vi "Calculate Color Index Array.vi"(8 "error in (no error)":errorcluster, 10 "3D Ribbon Datatype in":refnum<class "3D Ribbon Datatype.lvclass">, 11 "Plot Representation In":T1) -> (0 "error out":errorcluster, 2 "3D Ribbon Datatype out":refnum<class "3D Ribbon Datatype.lvclass">, 3 "Plot Representation Out":T1)   [LabVIEW 2017, in "3D Ribbon Datatype.lvclass"]
uses:
  <vilib>/Math Plots/3D Math Plots/3D Ribbon/3D Ribbon Datatype/3D Ribbon Datatype.lvclass
  <vilib>/Math Plots/3D Math Plots/3D Plot/3D Plot/Typedef/Plot Representation.ctl
  <vilib>/Math Plots/3D Math Plots/3D Plot/3D Plot/Typedef/Range Clusters.ctl
  <vilib>/Math Plots/3D Math Plots/3D Plot/3D Plot/Typedef/Mesh Data.ctl
  <vilib>/Math Plots/3D Math Plots/3D Ribbon/3D Ribbon Datatype/3D Ribbon Datatype.lvclass/3D Ribbon Datatype.ctl
  <vilib>/Math Plots/3D Math Plots/3D Plot/3D Plot Datatype/3D Plot Datatype.lvclass
  <vilib>/Math Plots/3D Math Plots/3D Plot/3D Plot/3D Plot.lvclass
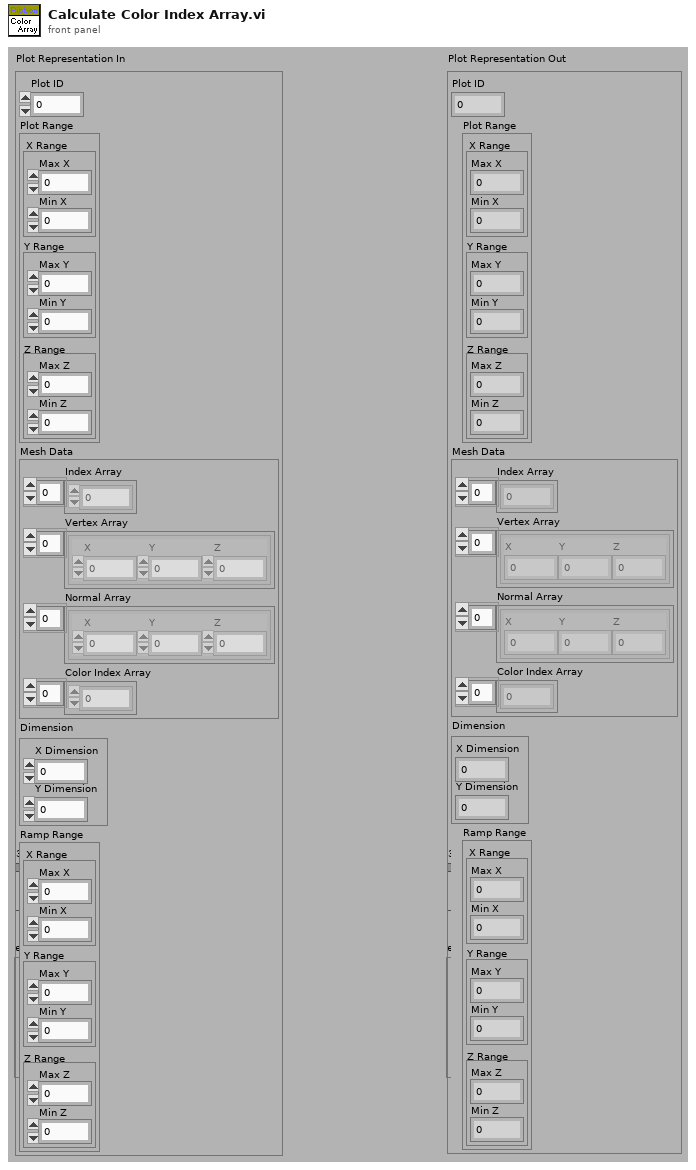
[diagram p1: front panel]
types:
  T1 = typedef "3D Plot.lvclass/Plot Representation.ctl" = cluster{"Plot ID":i32, "Plot Range":T2, "Mesh Data":T3, "Dimension":cluster{"X Dimension":i32, "Y Dimension":i32}, "Ramp Range":T2}
  T2 = typedef "3D Plot.lvclass/Range Clusters.ctl" = cluster{"X Range":cluster{"Max X":sgl, "Min X":sgl}, "Y Range":cluster{"Max Y":sgl, "Min Y":sgl}, "Z Range":cluster{"Max Z":sgl, "Min Z":sgl}}
  T3 = typedef "3D Plot.lvclass/Mesh Data.ctl" = cluster{"Index Array":u32[], "Vertex Array":cluster{"X":sgl, "Y":sgl, "Z":sgl}[], "Normal Array":cluster{"X":sgl, "Y":sgl, "Z":sgl}[], "Color Index Array":i32[]}
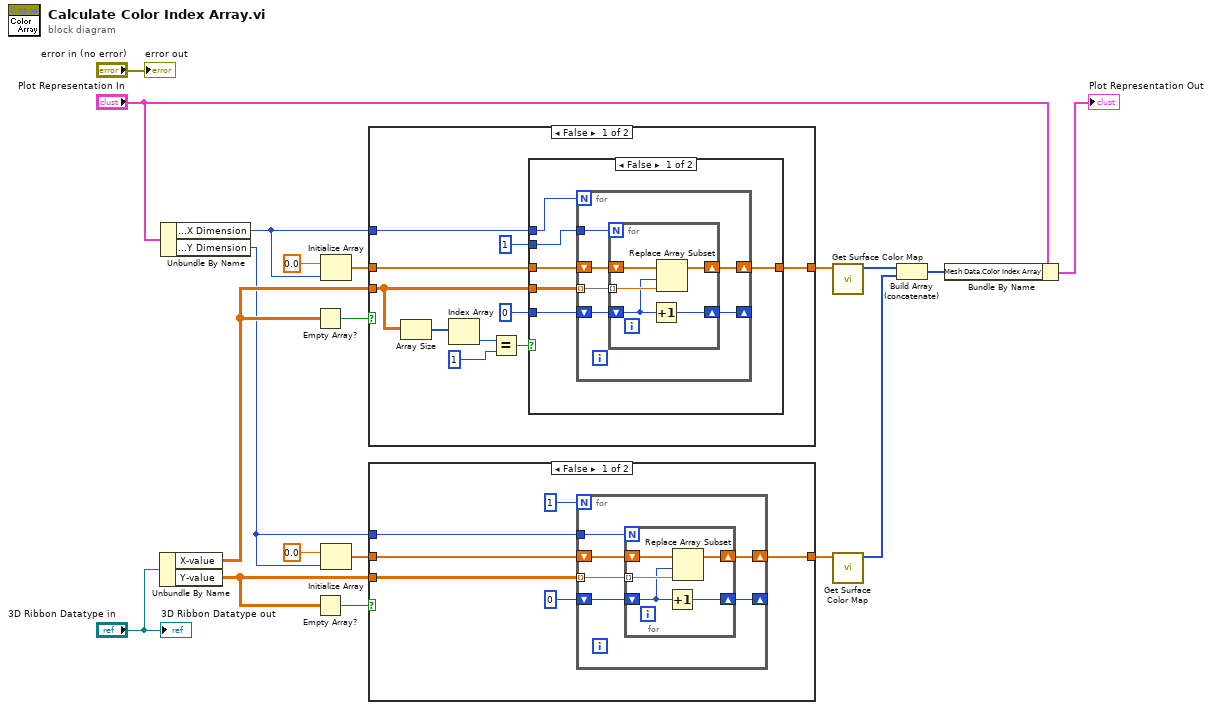
[diagram p0: block diagram]
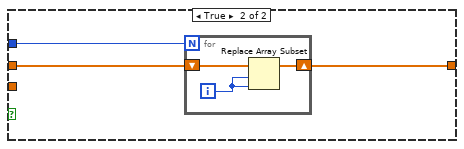
[diagram p2: hidden frame]
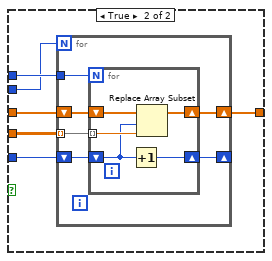
[diagram p3: hidden frame]
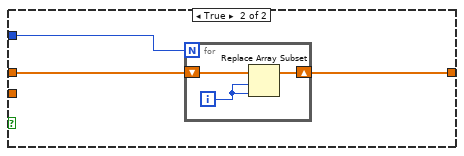
[diagram p4: hidden frame]
diagram:
  n1 = Unbundle By Name("3D Ribbon Datatype in") -> ("X-value"=w7:sgl[][], "Y-value"=w2:sgl[][])
  n2 = Unbundle By Name("Plot Representation In") -> ("Dimension.X Dimension"=w6:i32, "Dimension.Y Dimension"=w3:i32)
  n3 = Empty Array?(array=w7) -> (empty?=w10:bool)
  n4 = Empty Array?(array=w2) -> (empty?=w1:bool)
  n5 = Initialize Array(sgl 0.0 ("element"), w6) -> (w9:sgl[])
  n6 = Initialize Array(sgl 0.0 ("element"), w3) -> (w5:sgl[])
  n7 = case shown="False" w10 {
    tunnel: w9 -> [w29 w66]
    tunnel: [w28 w65] -> w8
    tunnel: w7 -> [w23 _]
    tunnel: w6 -> [w24 w64]
    frame False {
      n8 = Array Size(array=w23) -> (size(s)=w27:i32[])
      n9 = Index Array(array=w27) -> (element=w25:i32)  [unwired: 1 in]
      n10 = Equal?(x=w25, y=1 ("x")) -> (x = y?=w22:bool)
      n11 = case shown="False" w22 {
        tunnel: w29 -> [w35 w52]
        tunnel: [w34 w51] -> w28
        tunnel: w24 -> [w32 w50]
        tunnel: w23 -> [w33 w49]
        tunnel: 1 -> [w31 w48]
        tunnel: 0 -> [w30 w47]
        frame False {
          n12 = for {
            N: w32 -> [_]
            tunnel: w31 -> [w39]
            tunnel: w33 -> [w38] mode=indexing
            shift-right: [w40] -> w34
            shift-left: w35 -> [w41]
            shift-right: [w37] -> _
            shift-left: w30 -> [w36]
            n13 = for {
              N: w39 -> [_]
              shift-right: [w45] -> w40
              shift-left: w41 -> [w46]
              tunnel: w38 -> [w44] mode=indexing
              shift-right: [w43] -> w37
              shift-left: w36 -> [w42]
              n14 = Increment(x=w42) -> (x+1=w43:i32)
              n15 = Replace Array Subset(array=w46, new element=w44, index=w42) -> (w45:sgl[])
            }
          }
        }
        frame True {
          n16 = for {
            N: w48 -> [_]
            tunnel: w50 -> [w56]
            tunnel: w49 -> [w55] mode=indexing
            shift-right: [w57] -> w51
            shift-left: w52 -> [w58]
            shift-right: [w54] -> _
            shift-left: w47 -> [w53]
            n17 = for {
              N: w56 -> [_]
              shift-right: [w62] -> w57
              shift-left: w58 -> [w63]
              tunnel: w55 -> [w61] mode=indexing
              shift-right: [w60] -> w54
              shift-left: w53 -> [w59]
              n18 = Increment(x=w59) -> (x+1=w60:i32)
              n19 = Replace Array Subset(array=w63, new element=w61, index=w59) -> (w62:sgl[])
            }
          }
        }
      }
    }
    frame True {
      n20 = for {
        N: w64 -> [_]
        shift-right: [w68] -> w65
        shift-left: w66 -> [w69]
        i -> [w67]
        n21 = Replace Array Subset(array=w69, new element=w67, index=w67) -> (w68:sgl[])
      }
    }
  }
  n22 = case shown="False" w1 {
    tunnel: w5 -> [w75 w89]
    tunnel: [w74 w88] -> w4
    tunnel: w2 -> [w71 _]
    tunnel: w3 -> [w73 w87]
    frame False {
      n23 = for {
        N: 1 -> [_]
        tunnel: w73 -> [w79]
        shift-right: [w80] -> w74
        shift-left: w75 -> [w81]
        tunnel: w71 -> [w78] mode=indexing
        shift-right: [w77] -> _
        shift-left: 0 -> [w76]
        n24 = for {
          N: w79 -> [_]
          shift-right: [w85] -> w80
          shift-left: w81 -> [w86]
          tunnel: w78 -> [w84] mode=indexing
          shift-right: [w83] -> w77
          shift-left: w76 -> [w82]
          n25 = Increment(x=w82) -> (x+1=w83:i32)
          n26 = Replace Array Subset(array=w86, new element=w84, index=w82) -> (w85:sgl[])
        }
      }
    }
    frame True {
      n27 = for {
        N: w87 -> [_]
        shift-right: [w91] -> w88
        shift-left: w89 -> [w92]
        i -> [w90]
        n28 = Replace Array Subset(array=w92, new element=w90, index=w90) -> (w91:sgl[])
      }
    }
  }
  n29 = call <vilib>:"Get Surface Color Map.vi"("Amplifiy"=w8) -> ("Color Index Array"=w14:i32[])  [unwired: 1 in, 9 out]
  n30 = call <vilib>:"Get Surface Color Map.vi"("Amplifiy"=w4) -> ("Color Index Array"=w13:i32[])  [unwired: 1 in, 9 out]
  n31 = Build Array (concatenate)(w14, w13) -> (w12:i32[])
  n32 = Bundle By Name(cluster="Plot Representation In", "Mesh Data.Color Index Array"=w12) -> (→"Plot Representation Out":T1)
  "error out" <- "error in (no error)"
  "3D Ribbon Datatype out" <- "3D Ribbon Datatype in"
